vi "Automatic Target Selection.vi"(9 "Visible Objects [pix]":T2(array[cluster]), 10 "Scores":dbl[][](array[numeric]), 11 "Coords [um]":T3(array[cluster])) -> (1 "Stop":bool, 2 "Target OK":bool, 3 "Target Coordinates":T1)   [LabVIEW 2012, in "Targeting Unit.lvlib"]
uses:
  Targeting Unit.lvlib
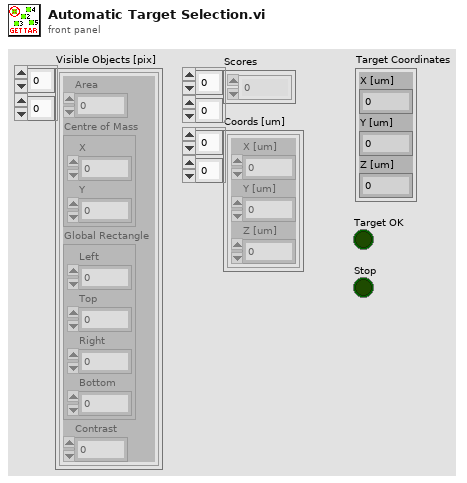
[diagram p1: front panel]
types:
  T1 = cluster{"X [um]":dbl, "Y [um]":dbl, "Z [um]":dbl}
  T2 = cluster{"Area":dbl, "Centre of Mass":cluster{"X":dbl, "Y":dbl}, "Global Rectangle":cluster{"Left":dbl, "Top":dbl, "Right":dbl, "Bottom":dbl}, "Contrast":dbl}[][]
  T3 = cluster{"X [um]":dbl, "Y [um]":dbl, "Z [um]":dbl}[][]
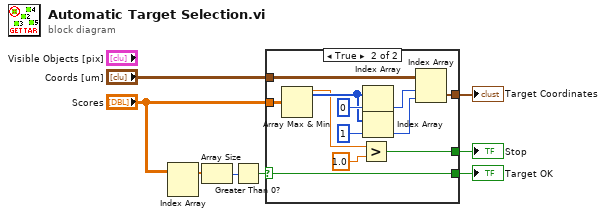
[diagram p0: block diagram]
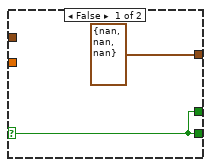
[diagram p2: hidden frame]
diagram:
  n1 = Index Array(array="Scores") -> (element=w2:dbl[])  [unwired: 2 in]
  n2 = Array Size(array=w2) -> (size(s)=w4:i32)
  n3 = Greater Than 0?(x=w4) -> (x > 0?=w3:bool)
  n4 = case shown="True" w3 {
    selector: w3 -> [w9 w14]
    tunnel: "Scores" -> [_ w22]
    tunnel: "Coords [um]" -> [_ w21]
    tunnel: [T1 {"X [um]"=nan, "Y [um]"=nan, "Z [um]"=nan} ("Target Coordinates") w15] -> w7
    tunnel: [w9 w14] -> w6
    tunnel: [w9 w11] -> w1
    frame False {
    }
    frame True {
      n5 = Array Max & Min(array=w22) -> (max value=w13:dbl, max index (indices)=w19:i32[])  [unwired: 2 out]
      n6 = Greater?(x=w13, y=1.0) -> (0:w11:bool)
      n7 = Index Array(array=w19, index=0) -> (element=w17:i32)
      n8 = Index Array(array=w19, index=1) -> (element=w16:i32)
      n9 = Index Array(array=w21, index (row)=w17, index (col)=w16) -> (element=w15:T1)
    }
  }
  "Target Coordinates" <- w7
  "Target OK" <- w6
  "Stop" <- w1
